vi "VisitLVArrayType.vi"(8 "error in (no error)":errorcluster, 10 "LVArrayType":refnum<class "LVArrayType.lvclass">, 11 "GetTypeAttributesVisitor in":refnum<class "GetTypeAttributesVisitor.lvclass">) -> (0 "error out":errorcluster, 3 "GetTypeAttributesVisitor out":refnum<class "GetTypeAttributesVisitor.lvclass">)   [LabVIEW 2020, in "Web Service Description.lvlib" / "GetTypeAttributesVisitor.lvclass"]
uses:
  <vilib>/AppBuilder/Engine/WebServiceDescription/GetTypeAttributesVisitor/GetTypeAttributesVisitor.lvclass
  <vilib>/AppBuilder/Engine/WebServiceDescription/LVDataTypes/LVArrayType/LVArrayType.lvclass
  e:/builds/penguin/labview/branches/2020/dev/dist/vi.lib/AppBuilder/Engine/WebServiceDescription/LVDataTypes/LVType/LVType.lvclass
  <vilib>/AppBuilder/Engine/WebServiceDescription/XMLGen/ValuePair.ctl
  <vilib>/AppBuilder/Engine/WebServiceDescription/GetTypeAttributesVisitor/GetTypeAttributesVisitor.lvclass/GetTypeAttributesVisitor.ctl
  <vilib>/AppBuilder/Engine/WebServiceDescription/XMLGen/XMLGen.lvlib
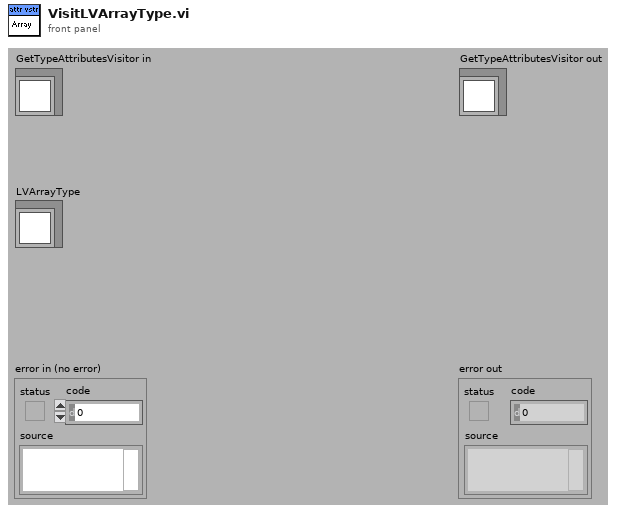
[diagram p1: front panel]
types:
  T1 = typedef "XMLGen.lvlib/ValuePair.ctl" = cluster{"Name":string, "Value":string}
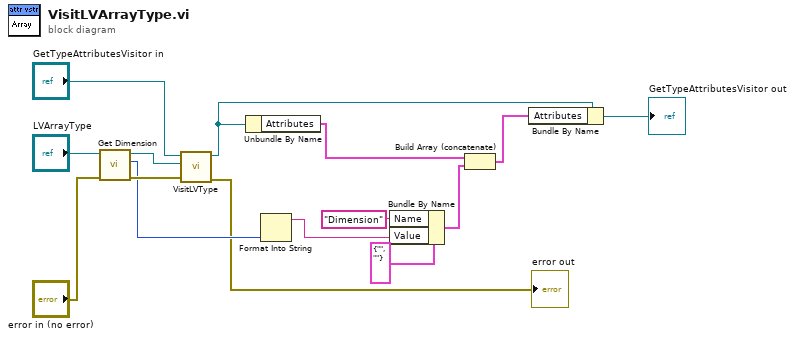
[diagram p0: block diagram]
diagram:
  n1 = call <vilib>:"Get Dimension.vi"("error in (no error)"="error in (no error)", "LVArrayType.lvclass in"="LVArrayType") -> ("error out"=w11:errorcluster, "Dimension"=w9:u32, "LVArrayType.lvclass out"=w10:refnum<class "LVArrayType.lvclass">)  [unwired: 7 out]
  n2 = call-dynamic "VisitLVType.vi"("error in (no error)"=w11, "LVType"=w10, "GetTypeAttributesVisitor in"="GetTypeAttributesVisitor in") -> ("error out"=→"error out":errorcluster, "GetTypeAttributesVisitor out"=w2:refnum<class "GetTypeAttributesVisitor.lvclass">)  [unwired: 7 out]
  n3 = Unbundle By Name(w2) -> ("Attributes"=w5:T1[])
  n4 = Format Into String(w9) -> (resulting string=w8:string)  [unwired: 3 in, 1 out]
  n5 = Bundle By Name(cluster=T1 {"Name"="", "Value"=""} ("Attribute"), "Name"="Dimension", "Value"=w8) -> (w4:T1)
  n6 = Build Array (concatenate)(w5, w4) -> (w3:T1[])
  n7 = Bundle By Name(cluster=w2, "Attributes"=w3) -> (→"GetTypeAttributesVisitor out":refnum<class "GetTypeAttributesVisitor.lvclass">)
